vi "as2_writeLogEntry.vi"(0 "Path In":path, 1 "Curr Param":dbl[](array[numeric])=[0.0, 3.0, 0.2, 1.0, 500.0] caption="Current Parameters", 2 "error in (no error)":errorcluster) -> (6 "error out":errorcluster)   [LabVIEW 2013]
uses:
  <vilib>/Utility/file.llb/Write To Spreadsheet File (string).vi
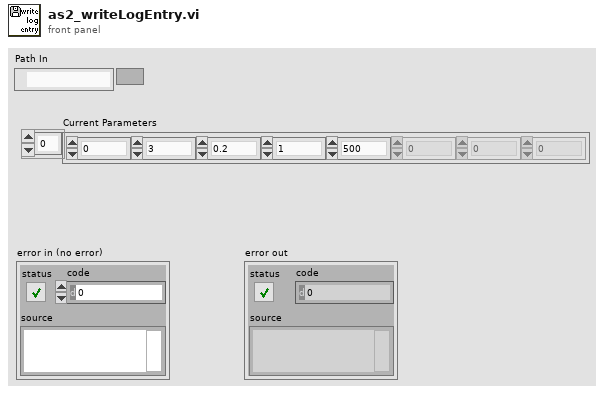
[diagram p1: front panel]
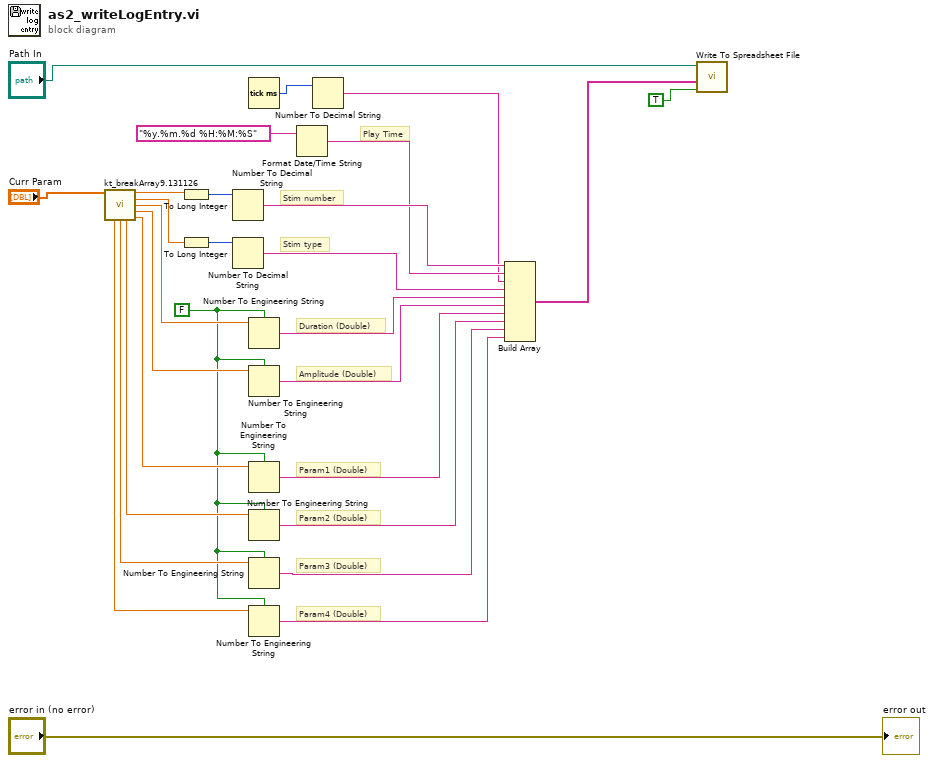
[diagram p0: block diagram]
diagram:
  w9 = FALSE ("use system decimal point (T)")
  # "Param4 (Double)"
  # "Param3 (Double)"
  # "Param2 (Double)"
  # "Param1 (Double)"
  # "Stim type"
  # "Amplitude (Double)"
  # "Duration (Double)"
  # "Play Time"
  # "Stim number"
  n1 = call "kt_breakArray9.131126.vi"("Current (or Cued Trial Parameters)"="Curr Param") -> ("Value 0"=w23:dbl, "Value 1"=w19:dbl, "Value 2"=w18:dbl, "Value 3"=w22:dbl, "Value 7"=w10:dbl, "Value 6"=w11:dbl, "Value 5"=w12:dbl, "Value 4"=w17:dbl)  [unwired: 6 in, 1 out]
  n2 = To Long Integer(number=w23) -> (32bit integer=w24:i32)
  n3 = To Long Integer(number=w19) -> (32bit integer=w21:i32)
  n4 = Number To Decimal String(number=w24) -> (decimal integer string=w4:string)  [unwired: 1 in]
  n5 = Number To Decimal String(number=w21) -> (decimal integer string=w20:string)  [unwired: 1 in]
  n6 = Tick Count (ms)() -> (millisecond timer value=w2:u32)
  n7 = Number To Engineering String(1:w9, 4:w18) -> (0:w16:string)  [unwired: 2 in]
  n8 = Number To Engineering String(1:w9, 4:w22) -> (0:w15:string)  [unwired: 2 in]
  n9 = Number To Engineering String(1:w9, 4:w17) -> (0:w7:string)  [unwired: 2 in]
  n10 = Number To Engineering String(1:w9, 4:w12) -> (0:w8:string)  [unwired: 2 in]
  n11 = Number To Engineering String(1:w9, 4:w11) -> (0:w6:string)  [unwired: 2 in]
  n12 = Number To Engineering String(1:w9, 4:w10) -> (0:w5:string)  [unwired: 2 in]
  n13 = Format Date/Time String(time format string (%c)="%y.%m.%d %H:%M:%S") -> (date/time string=w3:string)  [unwired: 2 in]
  n14 = Number To Decimal String(number=w2) -> (decimal integer string=w1:string)  [unwired: 1 in]
  n15 = Build Array(w4, w3, w1, w20, w16, w15, w7, w8, w6, w5) -> (w13:string[])
  n16 = call-poly <vilib>:"Write To Spreadsheet File.vi"("append to file? (new file:F)"=TRUE, "1D data"=w13, "file path (dialog if empty)"="Path In") -> ()  [unwired: 5 in, 1 out]
  "error out" <- "error in (no error)"
